vi "Remove_LDA_Spikes.vi"(3 "Current Block Number":i32, 4 "Analaysis info Cluster":T1={"Colour"=0, "Inst type"=enum."Pitot-static tube", "Inst name"="Manometer voltage", "Symbol"="U", "Code name"="", "Extra Info"="U", "Inst Array"=enum."PWA", "U"=0.0, "u^2"=0.0, "u^3"=0.0, "u^4"=0.0, "Skew_u"=0.0, "Kurt_u"=0.0, "Sd Error in Mean"=0.0, "% u'/U"=0.0, "X"=0.0, "Y"=0.0, "Z"=0.0, "Timescale integral Estimate"=0.0, "Sd Error in Variance"=0.0, "Calib File"=path "", "Calib Constants"=[], "Output Position"=FALSE, "Stats"=enum."None", "Av Sampling Rate"=0.0, "Av No of Samples"=0.0, "Total Meas Time (s)"=0.0, "OrigChName"="", "Max value"=0.0, "Min value"=0.0, "Req Sample Rate Hz"=0.0, "Sync Delay Time (s)"=0.0, "Ch No"=0, "Device"="", "Use Latest Calib"=FALSE, "Port"="", "Metadata Ch Names"=[], "Metadata Ch Values"=[], "Label"="", "chState"=enum."Solo", "Point Drift"=0.0, "inputConfig"=""} {"Kurt_u" format="%_3g"; "u^4" format="%_3g"; "u^3" format="%_3g"; "Sd Error in Variance" format="%_3g"; "u^2" format="%_3g"; "Sd Error in Mean" format="%_3g"; "U" format="%_3g"; "Sync Delay Time (s)" format="%.4f"; "Total Meas Time (s)" format="%_5g"; "Skew_u" format="%_3g"; "% u'/U" format="%_3g"}, 5 "Time (s) In":dbl[](array[numeric]), 6 "Time Trace In":T5) -> (0 "Time (s) Out":dbl[](array[numeric]), 1 "Analaysis info Cluster Out":T1={"Colour"=0, "Inst type"=enum."Pitot-static tube", "Inst name"="Manometer voltage", "Symbol"="U", "Code name"="", "Extra Info"="U", "Inst Array"=enum."PWA", "U"=0.0, "u^2"=0.0, "u^3"=0.0, "u^4"=0.0, "Skew_u"=0.0, "Kurt_u"=0.0, "Sd Error in Mean"=0.0, "% u'/U"=0.0, "X"=0.0, "Y"=0.0, "Z"=0.0, "Timescale integral Estimate"=0.0, "Sd Error in Variance"=0.0, "Calib File"=path "", "Calib Constants"=[], "Output Position"=FALSE, "Stats"=enum."None", "Av Sampling Rate"=0.0, "Av No of Samples"=0.0, "Total Meas Time (s)"=0.0, "OrigChName"="", "Max value"=0.0, "Min value"=0.0, "Req Sample Rate Hz"=0.0, "Sync Delay Time (s)"=0.0, "Ch No"=0, "Device"="", "Use Latest Calib"=FALSE, "Port"="", "Metadata Ch Names"=[], "Metadata Ch Values"=[], "Label"="", "chState"=enum."Solo", "Point Drift"=0.0, "inputConfig"=""} {"Kurt_u" format="%_3g"; "u^4" format="%_3g"; "u^3" format="%_3g"; "Sd Error in Variance" format="%_3g"; "u^2" format="%_3g"; "Sd Error in Mean" format="%_3g"; "U" format="%_3g"; "Sync Delay Time (s)" format="%.4f"; "Total Meas Time (s)" format="%_5g"; "Skew_u" format="%_3g"; "% u'/U" format="%_3g"}, 2 "Time trace Out":T5)   [LabVIEW 2022 SP3]
uses:
  <vilib>/Analysis/NI_AALBase.lvlib
  Controls/Resample mode.ctl
  Controls/Time_Trace_Cluster.ctl
  Controls/Inst_type.ctl
  Controls/Instrument_Array.ctl
  Controls/Analysis_info_cluster.ctl
  Controls/channelState.ctl
panel:
  out "After":cluster{"Time (s)":dbl[], "Eng Values":dbl[]}(graph)
  out "Before":cluster{"Time (s)":dbl[], "Eng Values":dbl[]}(graph)
  in  "Display plots":bool
  out "x-y":i32
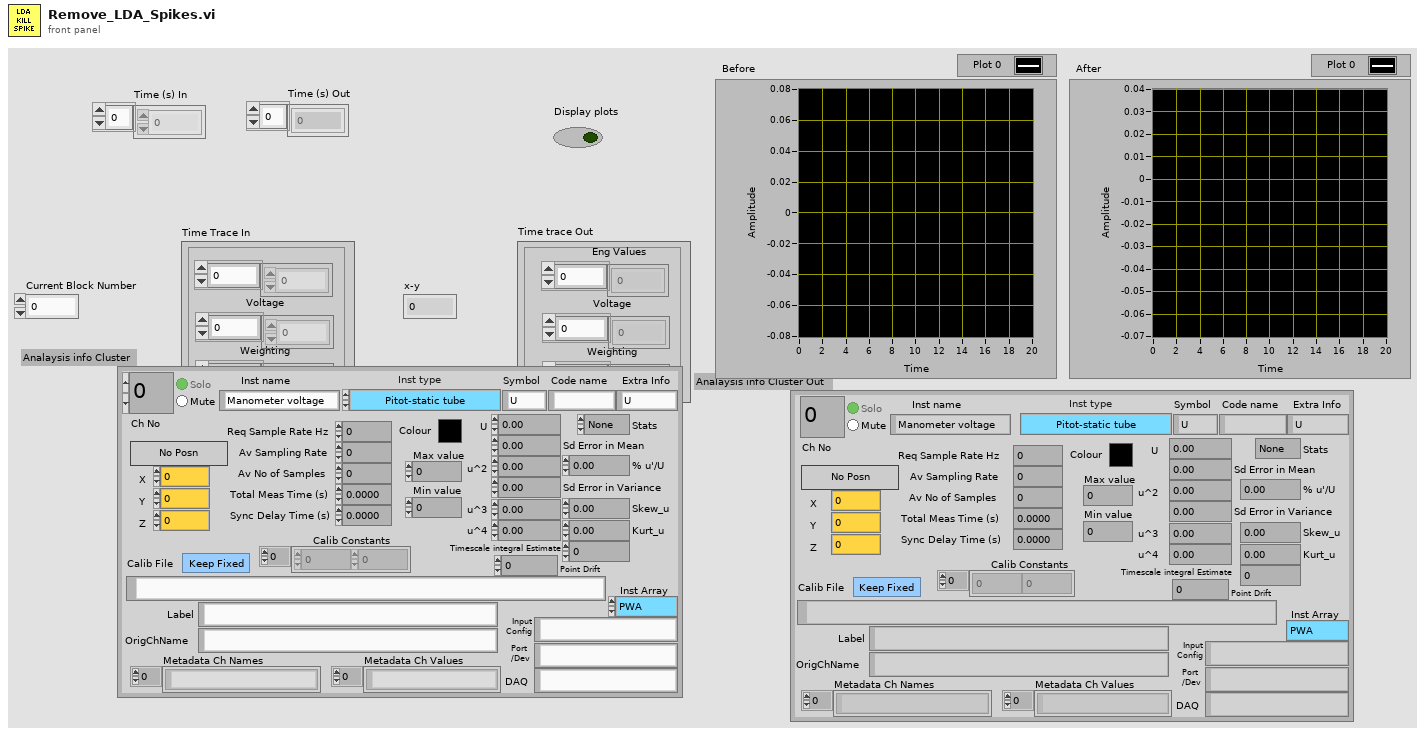
[diagram p1: front panel]
types:
  T1 = typedef "Analysis_info_cluster.ctl" = cluster{"Colour":u32, "Inst type":T2, "Inst name":string, "Symbol":string, "Code name":string, "Extra Info":string, "Inst Array":T3, "U":dbl, "u^2":dbl, "u^3":dbl, "u^4":dbl, "Skew_u":dbl, "Kurt_u":dbl, "Sd Error in Mean":dbl, "% u'/U":dbl, "X":dbl, "Y":dbl, "Z":dbl, "Timescale integral Estimate":dbl, "Sd Error in Variance":dbl, "Calib File":path, "Calib Constants":dbl[], "Output Position":bool, "Stats":enum16{"None", "Basic", "Full"}, "Av Sampling Rate":dbl, "Av No of Samples":dbl, "Total Meas Time (s)":dbl, "OrigChName":string, "Max value":dbl, "Min value":dbl, "Req Sample Rate Hz":dbl, "Sync Delay Time (s)":dbl, "Ch No":i16, "Device":string, "Use Latest Calib":bool, "Port":string, "Metadata Ch Names":string[], "Metadata Ch Values":string[], "Label":string, "chState":T4, "Point Drift":dbl, "inputConfig":string}
  T2 = typedef "Inst_type.ctl" = enum16{"Raw voltage", "Raw with zero offsetting", "Propeller anemometer", "Pressure Transducer", "Pitot-static tube", "Hot wire", "Cross wire 1", "Cross wire 2", "Generic Linear", "Generic Polynomial", "Generic BackPoly", "Fast FID", "Thermocouple", "Cold wire", "Pulsed Wire", "LDA Vel", "LDA Tran time", "LDA Arr time", "Microphone"}
  T3 = typedef "Instrument_Array.ctl" = enum16{"PWA", "LDA", "Analogue"}
  T4 = typedef "channelState.ctl" = enum32{"No Selection", "Solo", "Mute"}
  T5 = typedef "Time_Trace_Cluster.ctl" = cluster{"Weighting":dbl[], "Voltage":dbl[], "Eng Values":dbl[]}
  T6 = typedef "Resample mode.ctl" = cluster{"Mode":enum16{"Index", "Interpolate"}, "Index":dbl[]}
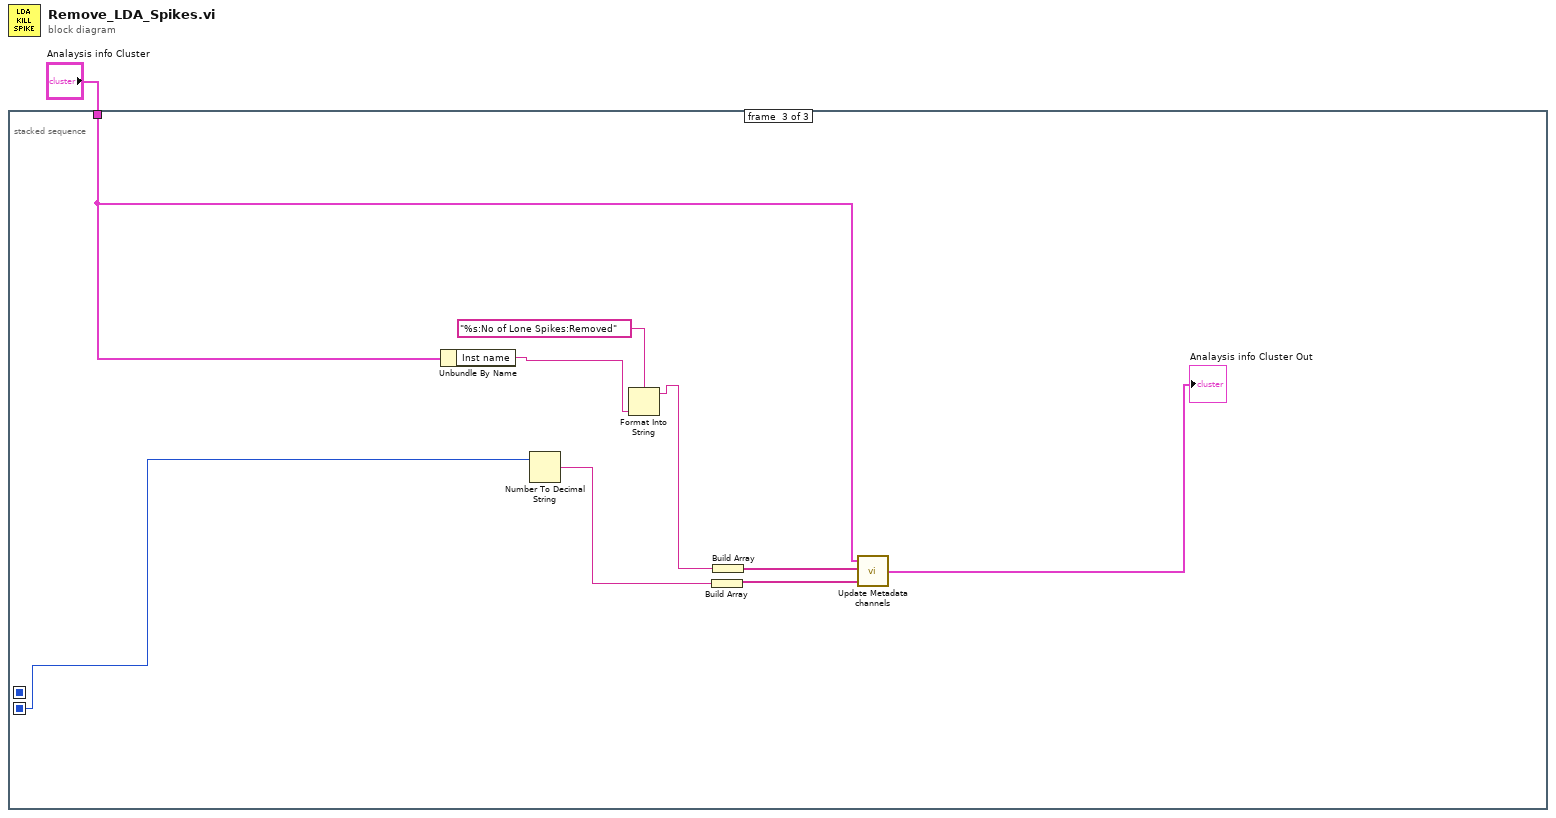
[diagram p0: block diagram]
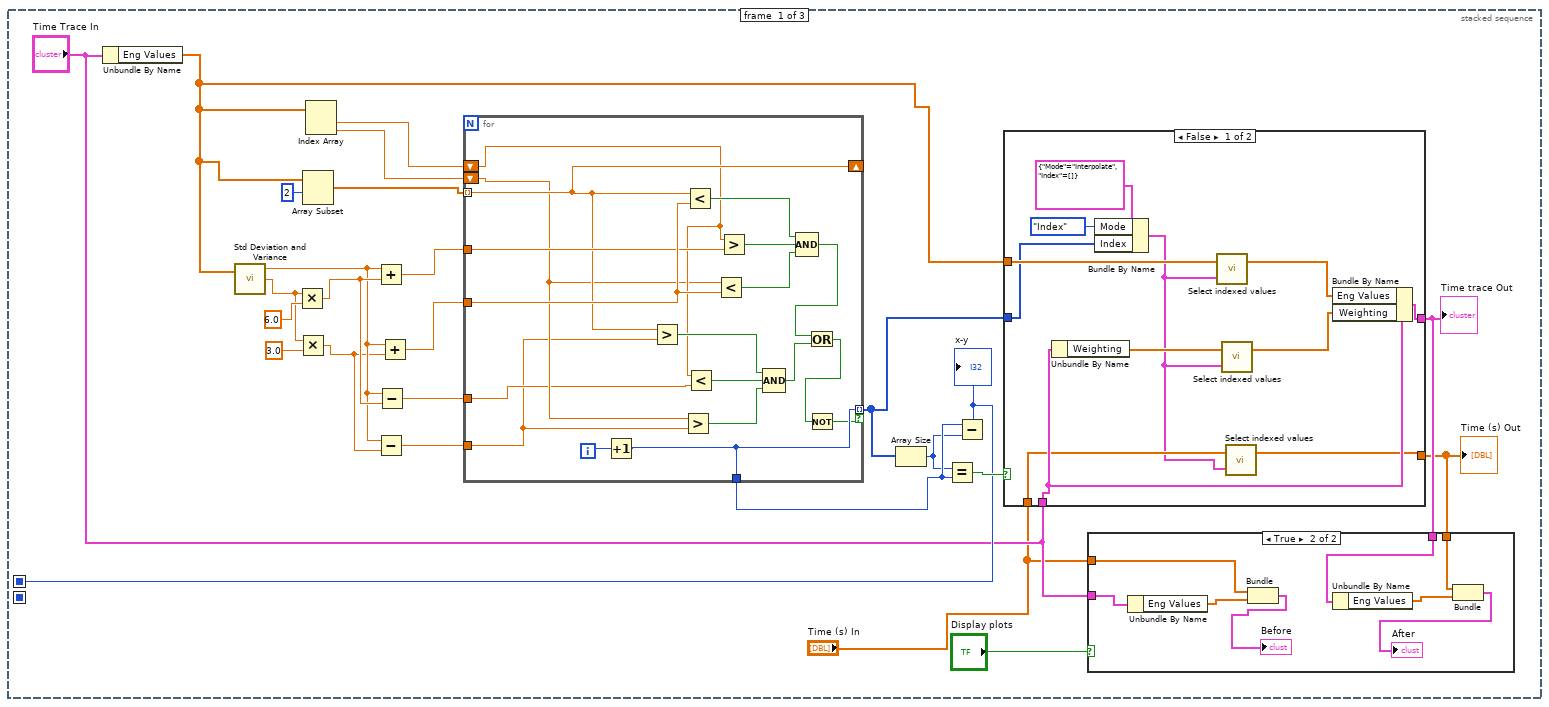
[diagram p2: hidden frame]
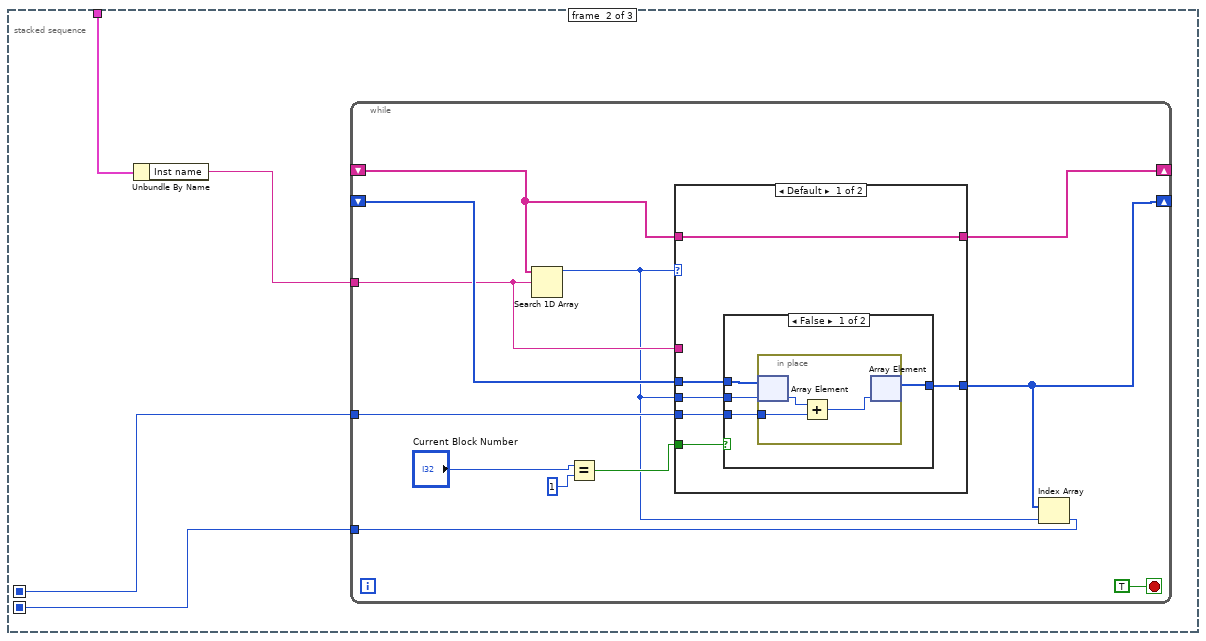
[diagram p5: hidden frame]
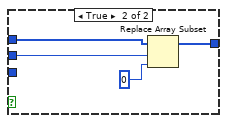
[diagram p6: hidden frame]
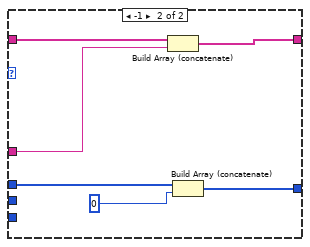
[diagram p7: hidden frame]
diagram:
  n1 = stacked-sequence {
    seq-local: [w12 _ _] -> [_ w71 _]
    seq-local: [_ w68 _] -> [_ _ w115]
    tunnel: "Analaysis info Cluster" -> [_ w70 w107]
    frame #0 {
      n2 = Unbundle By Name("Time Trace In") -> ("Eng Values"=w15:dbl[])
      n3 = call <vilib>:"Std Deviation and Variance.vi"("X"=w15) -> ("mean"=w10:dbl, "standard deviation"=w23:dbl)  [unwired: 1 in, 1 out]
      n4 = Multiply(x=w23, y=6.0) -> (x*y=w11:dbl)
      n5 = Multiply(x=w23, y=3.0) -> (x*y=w9:dbl)
      n6 = Array Subset(array=w15, index=2) -> (w18:dbl[])  [unwired: 1 in]
      n7 = Index Array(array=w15) -> (element #1=w21:dbl, element #2=w20:dbl)  [unwired: 2 in]
      n8 = Add(x=w10, y=w11) -> (x+y=w25:dbl)
      n9 = Subtract(x=w10, y=w9) -> (x-y=w7:dbl)
      n10 = Subtract(x=w10, y=w11) -> (x-y=w8:dbl)
      n11 = Add(x=w10, y=w9) -> (x+y=w22:dbl)
      n12 = for {
        tunnel: w25 -> [w66]
        tunnel: w18 -> [w57] mode=indexing
        shift-right: [w57] -> _
        shift-left: w21 -> [w56]
        shift-left: w20 -> [w55]
        tunnel: w22 -> [w67]
        tunnel: [w61] -> w16 mode=indexing if=w50
        tunnel: [w61] -> w14
        tunnel: w8 -> [w54]
        tunnel: w7 -> [w53]
        i -> [w62]
        n13 = Increment(x=w62) -> (x+1=w61:i32)
        n14 = Greater?(x=w57, y=w53) -> (0:w58:bool)
        n15 = Greater?(x=w55, y=w53) -> (0:w60:bool)
        n16 = Less?(x=w57, y=w67) -> (x < y?=w65:bool)
        n17 = Less?(x=w56, y=w54) -> (x < y?=w59:bool)
        n18 = Less?(x=w55, y=w67) -> (x < y?=w63:bool)
        n19 = Greater?(x=w56, y=w66) -> (0:w64:bool)
        n20 = Compound Arithmetic op=AND(w58, w59, w60) -> (w52:bool)
        n21 = Compound Arithmetic op=AND(w65, w64, w63) -> (w51:bool)
        n22 = Or(x=w51, y=w52) -> (x .or. y?=w49:bool)
        n23 = Not(x=w49) -> (.not. x?=w50:bool)
      }
      n24 = Array Size(array=w16) -> (size(s)=w13:i32)
      n25 = Equal?(x=w13, y=w14) -> (x = y?=w17:bool)
      n26 = Subtract(x=w14, y=w13) -> (x-y=w12:i32)
      "x-y" <- w12
      n27 = case shown="False" w17 {
        tunnel: [w45 w48] -> w4
        tunnel: "Time Trace In" -> [w46 w48]
        tunnel: w16 -> [w36 _]
        tunnel: w15 -> [w44 _]
        tunnel: "Time (s) In" -> [w40 w47]
        tunnel: [w39 w47] -> w2
        frame False {
          n28 = Unbundle By Name(w46) -> ("Weighting"=w42:dbl[])
          n29 = Bundle By Name(cluster=T6 {"Mode"=enum."Interpolate", "Index"=[]} ("Cluster"), "Mode"=enum16{"Index", "Interpolate"}."Index", "Index"=w36) -> (w35:T6)
          n30 = call "Select indexed values.vi"("Cluster"=w35, "Values"=w44) -> ("Values Out"=w43:dbl[])  [unwired: 1 in]
          n31 = call "Select indexed values.vi"("Cluster"=w35, "Values"=w42) -> ("Values Out"=w41:dbl[])  [unwired: 1 in]
          n32 = call "Select indexed values.vi"("Cluster"=w35, "Values"=w40) -> ("Values Out"=w39:dbl[])  [unwired: 1 in]
          n33 = Bundle By Name(cluster=w46, "Eng Values"=w43, "Weighting"=w41) -> (w45:T5)
        }
        frame True {
        }
      }
      "Time trace Out" <- w4
      "Time (s) Out" <- w2
      n34 = case shown="True" "Display plots" {
        tunnel: "Time Trace In" -> [_ w34]
        tunnel: w4 -> [_ w31]
        tunnel: "Time (s) In" -> [_ w28]
        tunnel: w2 -> [_ w27]
        frame False {
        }
        frame True {
          n35 = Unbundle By Name(w34) -> ("Eng Values"=w33:dbl[])
          n36 = Bundle("Time (s) In"=w28, "Eng Values"=w33) -> (→"Before":cluster{"Time (s) In":dbl[], "Eng Values":dbl[]})  [unwired: 1 in]
          n37 = Unbundle By Name(w31) -> ("Eng Values"=w32:dbl[])
          n38 = Bundle("Time (s) In"=w27, "Eng Values"=w32) -> (→"After":cluster{"Time (s) In":dbl[], "Eng Values":dbl[]})  [unwired: 1 in]
        }
      }
    }
    frame #1 {
      n39 = Unbundle By Name(w70) -> ("Inst name"=w69:string)
      n40 = while {
        tunnel: w69 -> [w79]
        shift-right: [w82] -> _
        shift-left: _ -> [w80]
        shift-right: [w74] -> _
        shift-left: _ -> [w81]
        tunnel: w71 -> [w77]
        tunnel: [w72] -> w68
        stop <- TRUE stop-if-true
        n41 = Search 1D Array(1D array=w80, element=w79) -> (index of element=w73:i32)  [unwired: 1 out]
        n42 = Equal?(x="Current Block Number", y=1) -> (x = y?=w75:bool)
        n43 = case shown="Default" w73 {
          tunnel: w80 -> [w89 w106]
          tunnel: w79 -> [_ w105]
          tunnel: [w89 w104] -> w82
          tunnel: w81 -> [w88 w103]
          tunnel: [w87 w102] -> w74
          tunnel: w73 -> [w86 _]
          tunnel: w75 -> [w85 _]
          tunnel: w77 -> [w84 _]
          frame Default {
            n44 = case shown="False" w85 {
              tunnel: w88 -> [w92 w100]
              tunnel: [w90 w99] -> w87
              tunnel: w86 -> [w93 w98]
              tunnel: w84 -> [w91 _]
              frame False {
                n45 = in-place {
                  in-place-border: w91 -> [w95]
                  n46 = in-place-array #1(w92, w93) -> (w96:i32)
                  n47 = Add(x=w96, y=w95) -> (x+y=w94:i32)
                  n48 = in-place-array #1(w94) -> (w90:i32[])  [unwired: 1 out]
                }
              }
              frame True {
                n49 = Replace Array Subset(array=w100, new element=0, index=w98) -> (w99:i32[])
              }
            }
          }
          frame -1 {
            n50 = Build Array (concatenate)(w106, w105) -> (w104:string[])
            n51 = Build Array (concatenate)(w103, 0) -> (w102:i32[])
          }
        }
        n52 = Index Array(array=w74, index=w73) -> (element=w72:i32)
      }
    }
    frame #2 {
      n53 = Unbundle By Name(w107) -> ("Inst name"=w113:string)
      n54 = Number To Decimal String(number=w115) -> (decimal integer string=w109:string)  [unwired: 1 out]
      n55 = Format Into String(format string="%s:No of Lone Spikes:Removed", w113) -> (resulting string=w108:string)  [unwired: 2 in, 1 out]
      n56 = Build Array(w109) -> (w111:string[])
      n57 = Build Array(w108) -> (w112:string[])
      n58 = call "Update Metadata channels.vi"("Metadata Values"=w111, "Metadata Names"=w112, "Analysis info Cluster in"=w107) -> ("Analysis info Cluster out"=→"Analaysis info Cluster Out":T1)
    }
  }
